vi "Read Actual Position.vi"(8 "error in (no error)":errorcluster, 11 "IgusMotorDrive in":refnum<class "IgusMotorDrive.lvclass">) -> (0 "error out":errorcluster, 1 "Response":T1={"Function Code"=1, "Data"=[], "RTU_DataBytes"=0} {"Data" format="%.0x"}, 2 "Command":T1={"Function Code"=1, "Data"=[], "RTU_DataBytes"=0} {"Data" format="%.0x"}, 3 "IgusMotorDrive out":refnum<class "IgusMotorDrive.lvclass">, 5 "Position":i32)   [LabVIEW 2016, in "IgusMotorDrive.lvclass"]
uses:
  IgusMotorDrive.lvclass
  typedefs/Statusword--enum.ctl
  Libraries/Modbus-Master/MB Master.lvlib
  Libraries/Modbus-Master/MB_Master_TCP/MB_Master_TCP.lvclass
  Libraries/Modbus-Master/MB_PDU/MB_PDU_Cluster.ctl
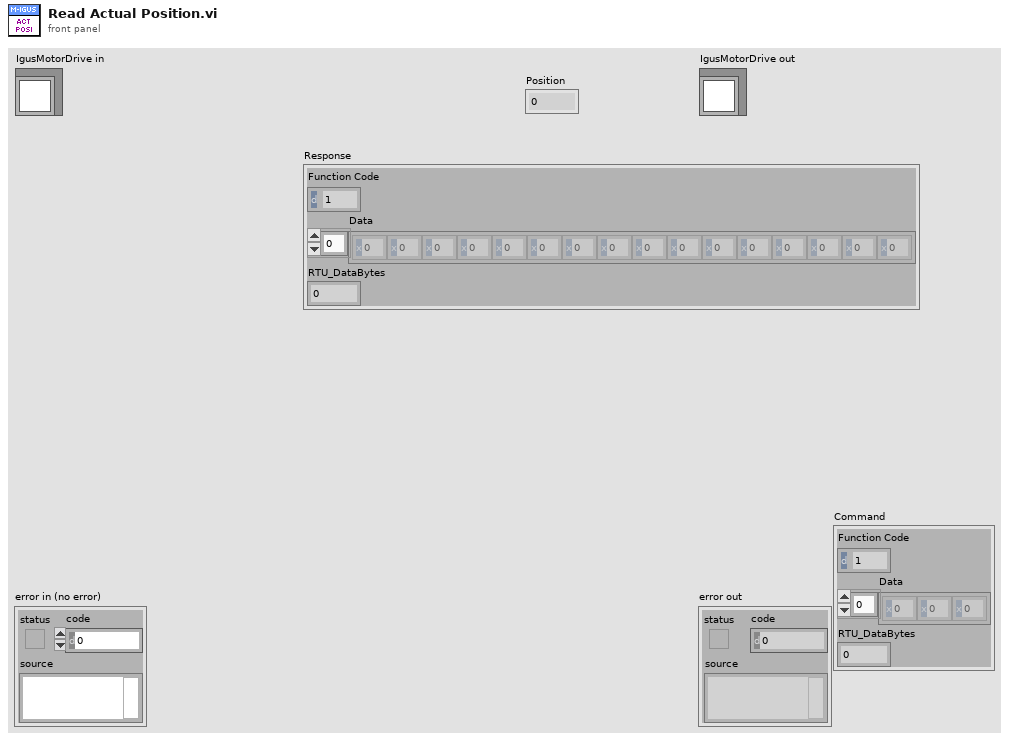
[diagram p1: front panel]
types:
  T1 = typedef "MB Master.lvlib/MB_PDU_Cluster.ctl" = cluster{"Function Code":u8, "Data":u8[], "RTU_DataBytes":i32}
  T2 = typedef "IgusMotorDrive.lvclass/Statusword--enum.ctl" = enum16{"Not Ready to Switch On", "Switch On Disabled", "Ready to Switch On", "Switched On", "Operation Enabled", "Quick Stop Active", "Fault Reaction Active", "Fault", "<Unknown>"}
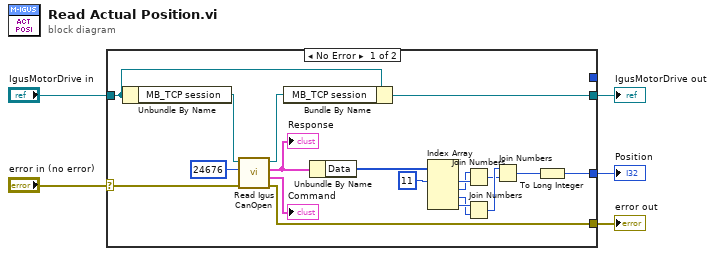
[diagram p0: block diagram]
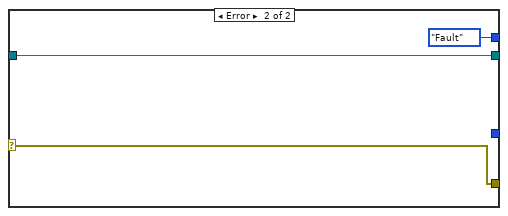
[diagram p2: hidden frame]
diagram:
  n1 = case shown="No Error" "error in (no error)" {
    selector: "error in (no error)" -> [w22 w27]
    tunnel: [w21 w27] -> w4
    tunnel: [w23 w26] -> w2
    tunnel: "IgusMotorDrive in" -> [w24 w26]
    tunnel: [_ Statusword--enum."Fault" ("Statusword")] -> _
    tunnel: [w6 _] -> w1
    frame No Error {
      n2 = Unbundle By Name(w24) -> ("MB_TCP session"=w20:refnum<class "MB_Master_TCP.lvclass">)
      n3 = call "Read Igus CanOpen.vi"("error in (no error)"=w22, "Address"=u16 24676, "MB session in"=w20) -> ("error out"=w21:errorcluster, "Command"=→"Command":T1, "Response"=w14:T1, "MB session out"=w19:refnum<class "MB_Master_TCP.lvclass">)  [unwired: 5 in]
      "Response" <- w14
      n4 = Bundle By Name(cluster=w24, "MB_TCP session"=w19) -> (w23:refnum<class "IgusMotorDrive.lvclass">)
      n5 = Unbundle By Name(w14) -> ("Data"=w18:u8[])
      n6 = Index Array(array=w18, index #1=11 ("index")) -> (element #1=w16:u8, element #2=w15:u8, element #3=w10:u8, element #4=w11:u8)  [unwired: 3 in]
      n7 = Join Numbers(hi=w15, lo=w16) -> ((hi.lo)=w8:u16)
      n8 = Join Numbers(hi=w11, lo=w10) -> ((hi.lo)=w9:u16)
      n9 = Join Numbers(hi=w9, lo=w8) -> ((hi.lo)=w7:u32)
      n10 = To Long Integer(number=w7) -> (32bit integer=w6:i32)
    }
    frame Error {
    }
  }
  "error out" <- w4
  "IgusMotorDrive out" <- w2
  "Position" <- w1
